vi "Measurement.vi"(8 "error in (no error)":errorcluster) -> (0 "error out":errorcluster, 2 "JSON object":string, 3 "sensors data":T1={"X"=0, "Y"=0, "Z"=0, "flame"=TRUE, "magnet"=FALSE, "obstacle"=FALSE, "sound"=[]})   [LabVIEW 2015]
uses:
  Sensors Data.ctl
  Device Packet.ctl
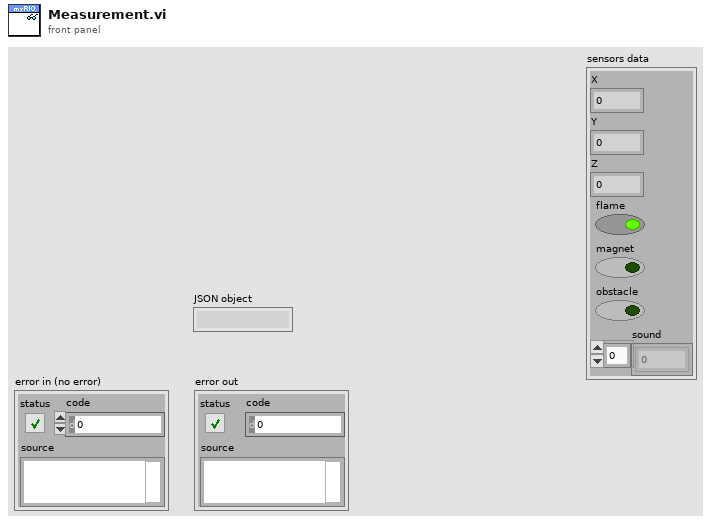
[diagram p1: front panel]
types:
  T1 = typedef "Sensors Data.ctl" = cluster{"X":i8, "Y":i8, "Z":i8, "flame":bool, "magnet":bool, "obstacle":bool, "sound":sgl[]}
  T2 = typedef "Device Packet.ctl" = cluster{"sensors data":T1}
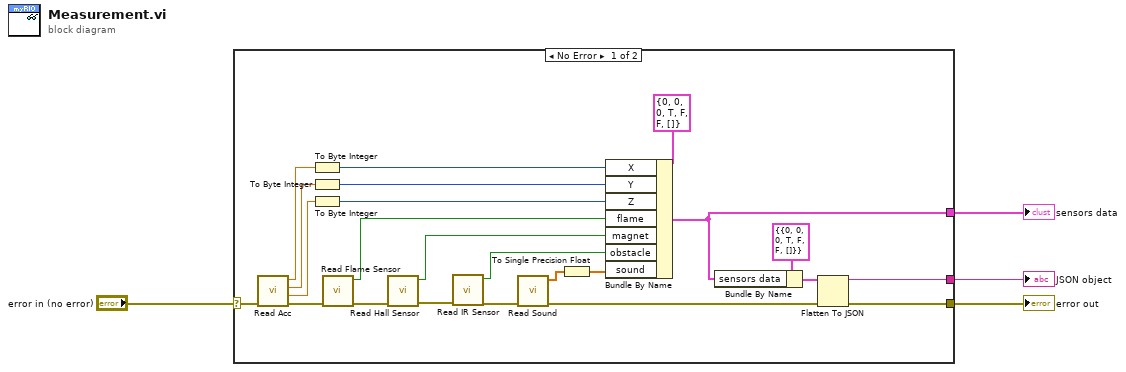
[diagram p0: block diagram]
diagram:
  n1 = case shown="No Error" "error in (no error)" {
    selector: "error in (no error)" -> [w12 w28]
    tunnel: [w18 _] -> w4
    tunnel: [w16 w28] -> w3
    tunnel: [w15 _] -> w1
    frame No Error {
      n2 = call "Read Acc.vi"("error in (no error)"=w12) -> ("error out"=w8:errorcluster, "Z"=w22:dbl, "Y"=w24:dbl, "X"=w27:dbl)  [unwired: 7 in]
      n3 = To Byte Integer(number=w27) -> (8bit integer=w25:i8)
      n4 = To Byte Integer(number=w24) -> (8bit integer=w23:i8)
      n5 = To Byte Integer(number=w22) -> (8bit integer=w21:i8)
      n6 = call "Read Flame Sensor.vi"("error in (no error)"=w8) -> ("error out"=w7:errorcluster, "flame detected?"=w20:bool)  [unwired: 9 in]
      n7 = call "Read Hall Sensor.vi"("error in (no error)"=w7) -> ("error out"=w6:errorcluster, "Yeah Bitch!! Magnets!!"=w10:bool)  [unwired: 9 in]
      n8 = call "Read IR Sensor.vi"("error in (no error)"=w6) -> ("error out"=w5:errorcluster, "obstacle detected?"=w9:bool)  [unwired: 9 in]
      n9 = call "Read Sound.vi"("error in (no error)"=w5) -> ("error out"=w11:errorcluster, "sound"=w14:dbl[])  [unwired: 9 in]
      n10 = To Single Precision Float(number=w14) -> (single precision float=w13:sgl[])
      n11 = Bundle By Name(cluster=T1 {"X"=0, "Y"=0, "Z"=0, "flame"=TRUE, "magnet"=FALSE, "obstacle"=FALSE, "sound"=[]}, "X"=w25, "Y"=w23, "Z"=w21, "flame"=w20, "magnet"=w10, "obstacle"=w9, "sound"=w13) -> (w18:T1)
      n12 = Bundle By Name(cluster=T2 {"sensors data"={"X"=0, "Y"=0, "Z"=0, "flame"=TRUE, "magnet"=FALSE, "obstacle"=FALSE, "sound"=[]}} ("d"), "sensors data"=w18) -> (w17:T2)
      n13 = Flatten To JSON(anything=w17, error in (no error)=w11) -> (JSON string=w15:string, 11:w16:errorcluster)  [unwired: 1 in]
    }
    frame Error {
    }
  }
  "error out" <- w3
  "JSON object" <- w1
  "sensors data" <- w4
